vi "Setup.vi"(11 "Connection Handler in":refnum<class "Connection Handler.lvclass">) -> (3 "Connection Handler out":refnum<class "Connection Handler.lvclass">)   [LabVIEW 2017, in "Network Interface.lvlib" / "Connection Handler.lvclass"]
uses:
  <vilib>/gpm_packages/@cs/Network-sink/Source/Network Interface/Connection Handler/Connection Handler.lvclass
  <vilib>/gpm_packages/@cs/Network-sink/Source/Network Interface/Message Queue/Message Queue.lvclass/Message Queue.ctl
  <vilib>/gpm_packages/@cs/Network-sink/Source/Network Interface/Connection Handler/Connection Handler.lvclass/Connection Handler.ctl
  <vilib>/gpm_packages/@cs/Network-sink/Source/Network Interface/Connection Handler/Message Names ENUM.ctl
  f04b9c6f-ea97-43db-ada0-b6a62c813008.vi
  <vilib>/gpm_packages/@cs/Network-sink/Source/Network Interface/Message Queue/Protected Enqueue.vi
  <vilib>/gpm_packages/@cs/Network-sink/Source/Network Interface/Message Queue/Message Queue.lvclass
  <vilib>/gpm_packages/@cs/Network-sink/Source/Network Interface/IConnection/IConnection.lvclass
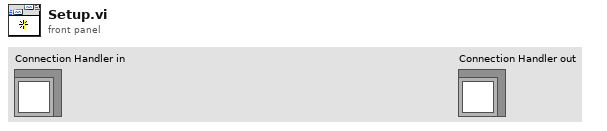
[diagram p1: front panel]
types:
  T1 = typedef "Network Interface.lvlib/Connection Handler.lvclass/Message Names ENUM.ctl" = enum16{"Transmit Message", "Stop"}
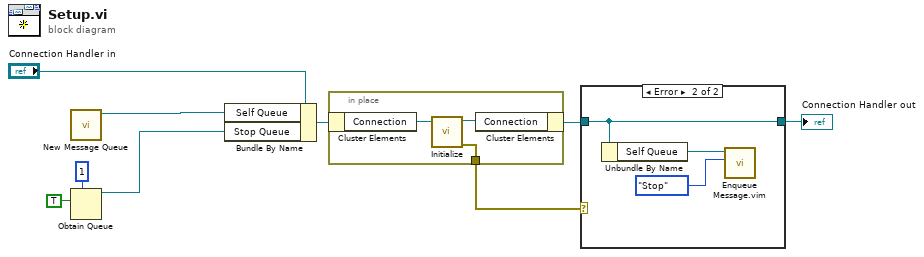
[diagram p0: block diagram]
diagram:
  n1 = call <vilib>:"New Message Queue.vi"() -> ("Message Queue out"=w5:refnum<class "Message Queue.lvclass">)  [unwired: 10 in, 1 out]
  n2 = Obtain Queue(max queue size (-1, unlimited)=1, element data type=TRUE) -> (queue out=w6:refnum<queue>)  [unwired: 3 in, 2 out]
  n3 = Bundle By Name(cluster="Connection Handler in", "Self Queue"=w5, "Stop Queue"=w6) -> (w4:refnum<class "Connection Handler.lvclass">)
  n4 = in-place {
    in-place-border: [w10] -> w1
    n5 = in-place-cluster #1(w4) -> ("Connection"=w12:refnum<class "IConnection.lvclass">)
    n6 = call-dynamic "Initialize.vi"("IConnection in"=w12) -> ("error out"=w10:errorcluster, "IConnection out"=w11:refnum<class "IConnection.lvclass">)  [unwired: 9 in]
    n7 = in-place-cluster #1("Connection"=w11) -> (w3:refnum<class "Connection Handler.lvclass">)
  }
  n8 = case shown="Error" w1 {
    tunnel: [w13 w15] -> w2
    tunnel: w3 -> [w13 w15]
    frame No Error {
    }
    frame Error {
      n9 = Unbundle By Name(w15) -> ("Self Queue"=w16:refnum<class "Message Queue.lvclass">)
      n10 = call "Enqueue Message.vim"("Msg"=Message_Names_ENUM."Stop", "Message Queue in"=w16) -> ()  [unwired: 8 in, 2 out]
    }
  }
  "Connection Handler out" <- w2
